vi "Scale Single.vi"(6 "Variable Configuration":T1[](array[typedef]) {"Scaling"."Offset" format="%.5f"; "Scaling"."Gain" format="%.5f"; "Limits and responces"."Limits"."H" format="%.3f"; "Limits and responces"."Limits"."L" format="%.3f"; "Limits and responces"."Limits"."HH" format="%.3f"; "Limits and responces"."Limits"."LL" format="%.3f"}, 10 "Unscaled data in":dbl, 11 "Var Tag":u16) -> (2 "Scaled data out":dbl)   [LabVIEW 2011]
doc: "This VI scales a waveform. The data buffer only provides unscaled data and hence this VI is necessary."
uses:
  User Setting Analog Channel Bg.ctl
  Scaling.ctl
  Alarm Setup Analog.ctl
  Alarm Responce.ctl
  Action List.ctl
  Limits.ctl
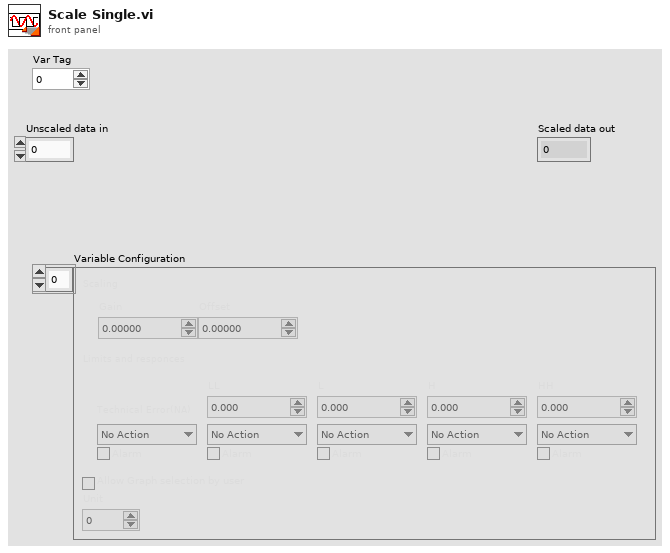
[diagram p1: front panel]
types:
  T1 = typedef "User Setting Analog Channel Bg.ctl" = cluster{"Scaling":T2, "Limits and responces":T3, "Allow Graph selection by user":bool, "Unit":u16}
  T2 = typedef "Scaling.ctl" = cluster{"Gain":dbl, "Offset":dbl}
  T3 = typedef "Alarm Setup Analog.ctl" = cluster{"Technical Error(NA)":T4, "LL":T4, "L":T4, "H":T4, "HH":T4, "Limits":T6}
  T4 = typedef "Alarm Responce.ctl" = cluster{"Action":T5, "Alarm":bool}
  T5 = typedef "Action List.ctl" = enum16{"No Action", "Stop Motor", "Turn Off HV"}
  T6 = typedef "Limits.ctl" = cluster{"LL":dbl, "L":dbl, "H":dbl, "HH":dbl}
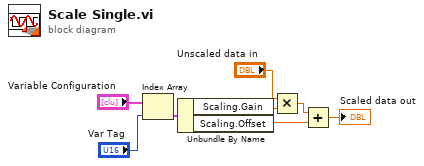
[diagram p0: block diagram]
diagram:
  n1 = Index Array(array="Variable Configuration", index="Var Tag") -> (element=w6:T1)
  n2 = Unbundle By Name(w6) -> ("Scaling.Gain"=w5:dbl, "Scaling.Offset"=w4:dbl)
  n3 = Multiply(x="Unscaled data in", y=w5) -> (x*y=w7:dbl)
  n4 = Add(x=w7, y=w4) -> (x+y=→"Scaled data out":dbl)
